vi "Real Time.vi"() -> ()   [LabVIEW 2016]
uses:
  <vilib>/Platform/TimedLoop/XDataNode/timing_clust.ctl
  <vilib>/Platform/TimedLoop/XDataNode/nitl_modes.ctl
  <vilib>/Platform/TimedLoop/XDataNode/wakeup.ctl
  <vilib>/FPGAPlugInAG/sbRIO-9636/niLvFpga_Open_sbRIO-9636.vi
  <vilib>/rvi/interface/common/dynamic/niFpgaDynamicAddResources.vi
  <vilib>/Utility/error.llb/Error Cluster From Error Code.vi
  <vilib>/rvi/errors/niLvFpgaAdjustHostInterfaceError.vi
  <vilib>/FPGAPlugInAG/Dynamic/niLvFpga_Close_Dynamic.vi
  <vilib>/Platform/TimedLoop/XDataNode/XDataNode.xnode
  <vilib>/rvi/interface/nirviOpenFPGA/nirviOpenFPGA.xnode
  FPGA Bitfiles/Practice_FPGATarget_GrapheneFlexionT_17S50-wD-zg.lvbitx
  Graphene Flexion Test.vi
  <vilib>/rvi/interface/nirviReadWriteControl/nirviReadWriteControl.xnode
  <vilib>/rvi/interface/nirviCloseFPGA/nirviCloseFPGA.xnode
  <vilib>/Platform/TimedLoop/XDataNode/XDNodeRunTimeDep.lvlib
  NiFpgaLv.dll
  <vilib>/rvi/interface/Simulation/niFpgaSimulationCallBeginRW.vi
panel:
  out "1Hz Output 3":dbl(graph)
  out "0.5Hz Output 2":dbl(graph)
  out "0.75Hz Output":dbl(graph)
  out "Unfiltered Output":sgl(graph)
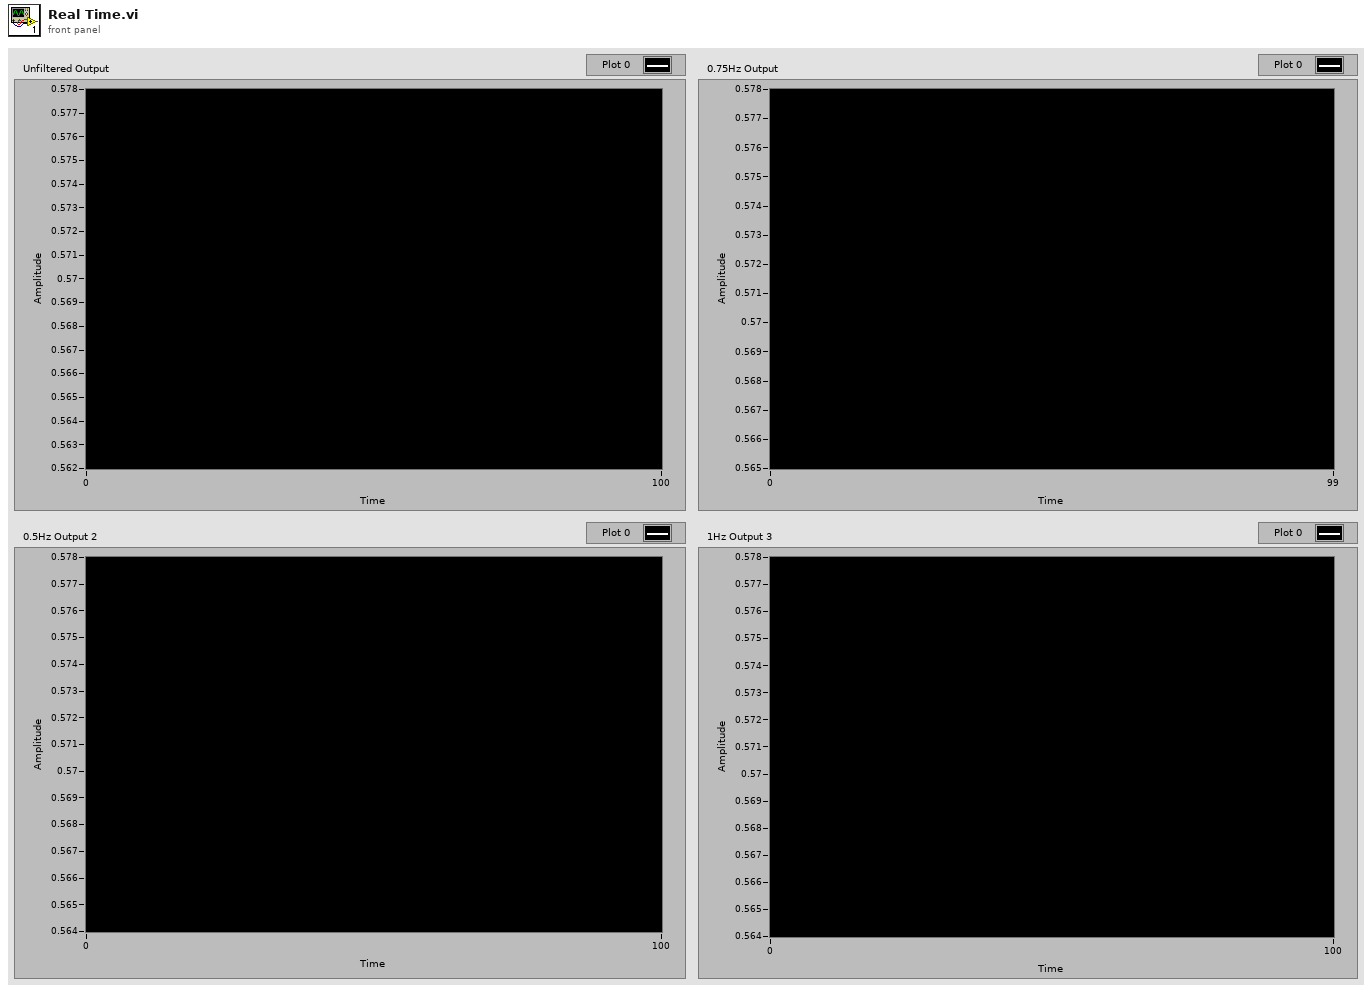
[diagram p1: front panel]
types:
  T1 = typedef "XDNodeRunTimeDep.lvlib/timing_clust.ctl" = cluster{"Expected End [f-1]":u64, "Actual End [f-1]":u64, "Finished Late? [f-1]":bool, "Expected End [i-1]":u64, "Actual End [i-1]":u64, "Finished Late? [i-1]":bool, "Expected Start [i]":u64, "Actual Start [i]":u64, "Expected Start [f]":u64, "Actual Start [f]":u64, "Source Name":string, "Structure Name":string, "Period":i64, "Deadline":i64, "Offset":i64, "Start":i64, "Priority":i32, "Timeout":i32, "Mode":T2, "Wakeup Reason":T3, "Error":errorcluster, "Source Type":string, "Secondary Source Type":string, "Global End Time":u64, "Global Start Time":u64, "Frame Duration":u64, "Iteration Duration":u64, "Assigned CPU":i32, "I/O Scan Engine Mode":u32}
  T2 = typedef "XDNodeRunTimeDep.lvlib/nitl_modes.ctl" = enum32{"No Change", "Process missed periods, maintain original phase", "Discard missed periods, maintain original phase", "Process missed periods, ignore original phase", "Discard missed periods, ignore original phase"}
  T3 = typedef "XDNodeRunTimeDep.lvlib/wakeup.ctl" = enum32{"Normal", "Aborted", "Asynchronous wakeup", "Timing source error", "Timed loop error", "Timeout"}
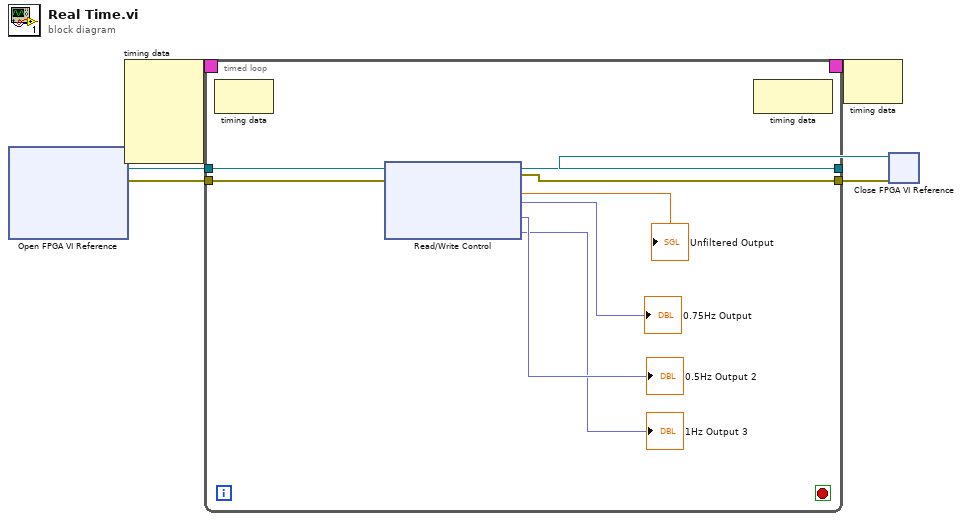
[diagram p0: block diagram]
diagram:
  n1 = xnode "Open FPGA VI Reference"() -> ("FPGA VI Reference Out"=w1:refnum<k20>, "error out"=w2:errorcluster)  [unwired: 2 in]
  n2 = node-c288() -> (w6:T1)  [unwired: 5 in]
  n3 = timed-loop {
    timing: w6 -> [_]
    timing-out: [_] -> w5
    tunnel: w1 -> [w11]
    tunnel: w2 -> [w10]
    tunnel: [w14] -> w4
    tunnel: [w13] -> w3
    stop <- _ stop-if-true
    n4 = node-c288() -> ()  [unwired: 1 in, 1 out]
    n5 = xnode "Read/Write Control"("FPGA VI Reference In"=w11, "error in"=w10) -> ("FPGA VI Reference Out"=w14:refnum<k20>, "error out"=w13:errorcluster, "Unfiltered Signal"=→"Unfiltered Output":sgl, "Filtered Signal 0.75Hz"=→"0.75Hz Output":fxp<+/-,28,9>, "Filtered Signal 0.500Hz"=→"0.5Hz Output 2":fxp<+/-,28,9>, "Filtered Signal 1Hz"=→"1Hz Output 3":fxp<+/-,28,9>)
    n6 = node-c288() -> ()  [unwired: 1 in, 1 out]
  }
  n7 = node-c288(w5) -> ()  [unwired: 1 out]
  n8 = xnode "Close FPGA VI Reference"("FPGA VI Reference In"=w4, "error in"=w3) -> ()  [unwired: 1 out]
